vi "Bezier Spline.vi"(6 "positions":cluster{dbl[]}[](array[cluster]), 7 "Turn Rate":dbl=5.0 format="%#_13g", 8 "ending orientation (deg)":sgl=nan, 9 "starting orientation (deg)":sgl=nan, 10 "percision":sgl=0.01, 11 "waypts":cluster{"x":sgl, "y":sgl}[](array[cluster])) -> (0 "cubic spline ctrl pts":cluster{sgl, sgl}[][](array[cluster]), 1 "Tangents":cluster{sgl, sgl}[](array[cluster]), 2 "ctrl pts":cluster{sgl, sgl}[][](array[cluster]), 3 "bezier spline":cluster{"curve ":T1}[](array[cluster]), 4 "position out":sgl[][](array[numeric]))   [LabVIEW 2025]
uses:
  Types/Bezier Curve.ctl
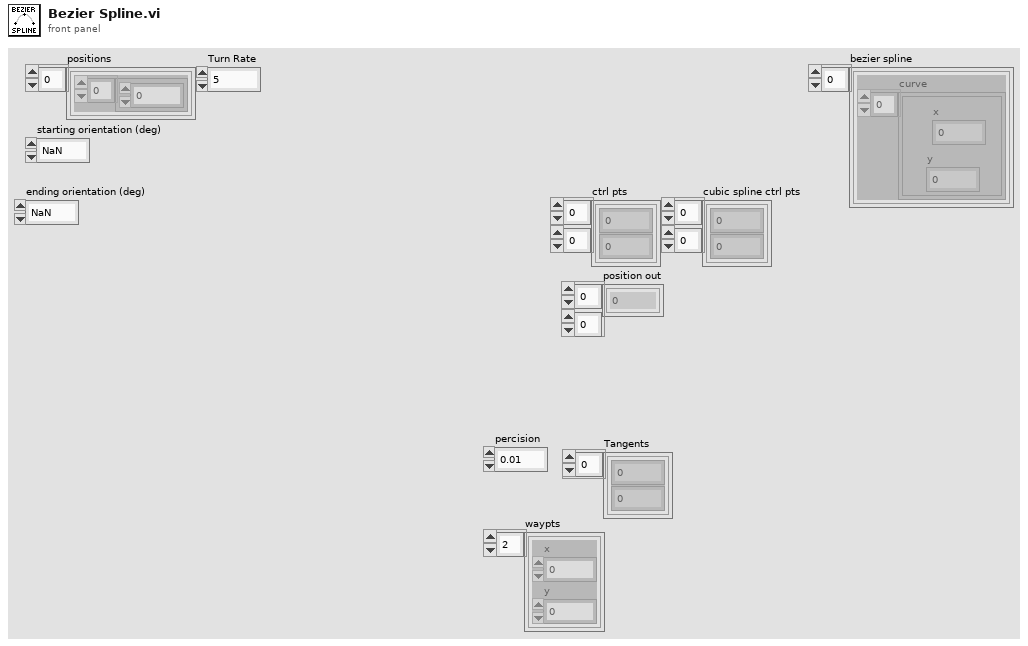
[diagram p1: front panel]
types:
  T1 = typedef "Bezier Curve.ctl" = cluster{"x":sgl, "y":sgl}[]
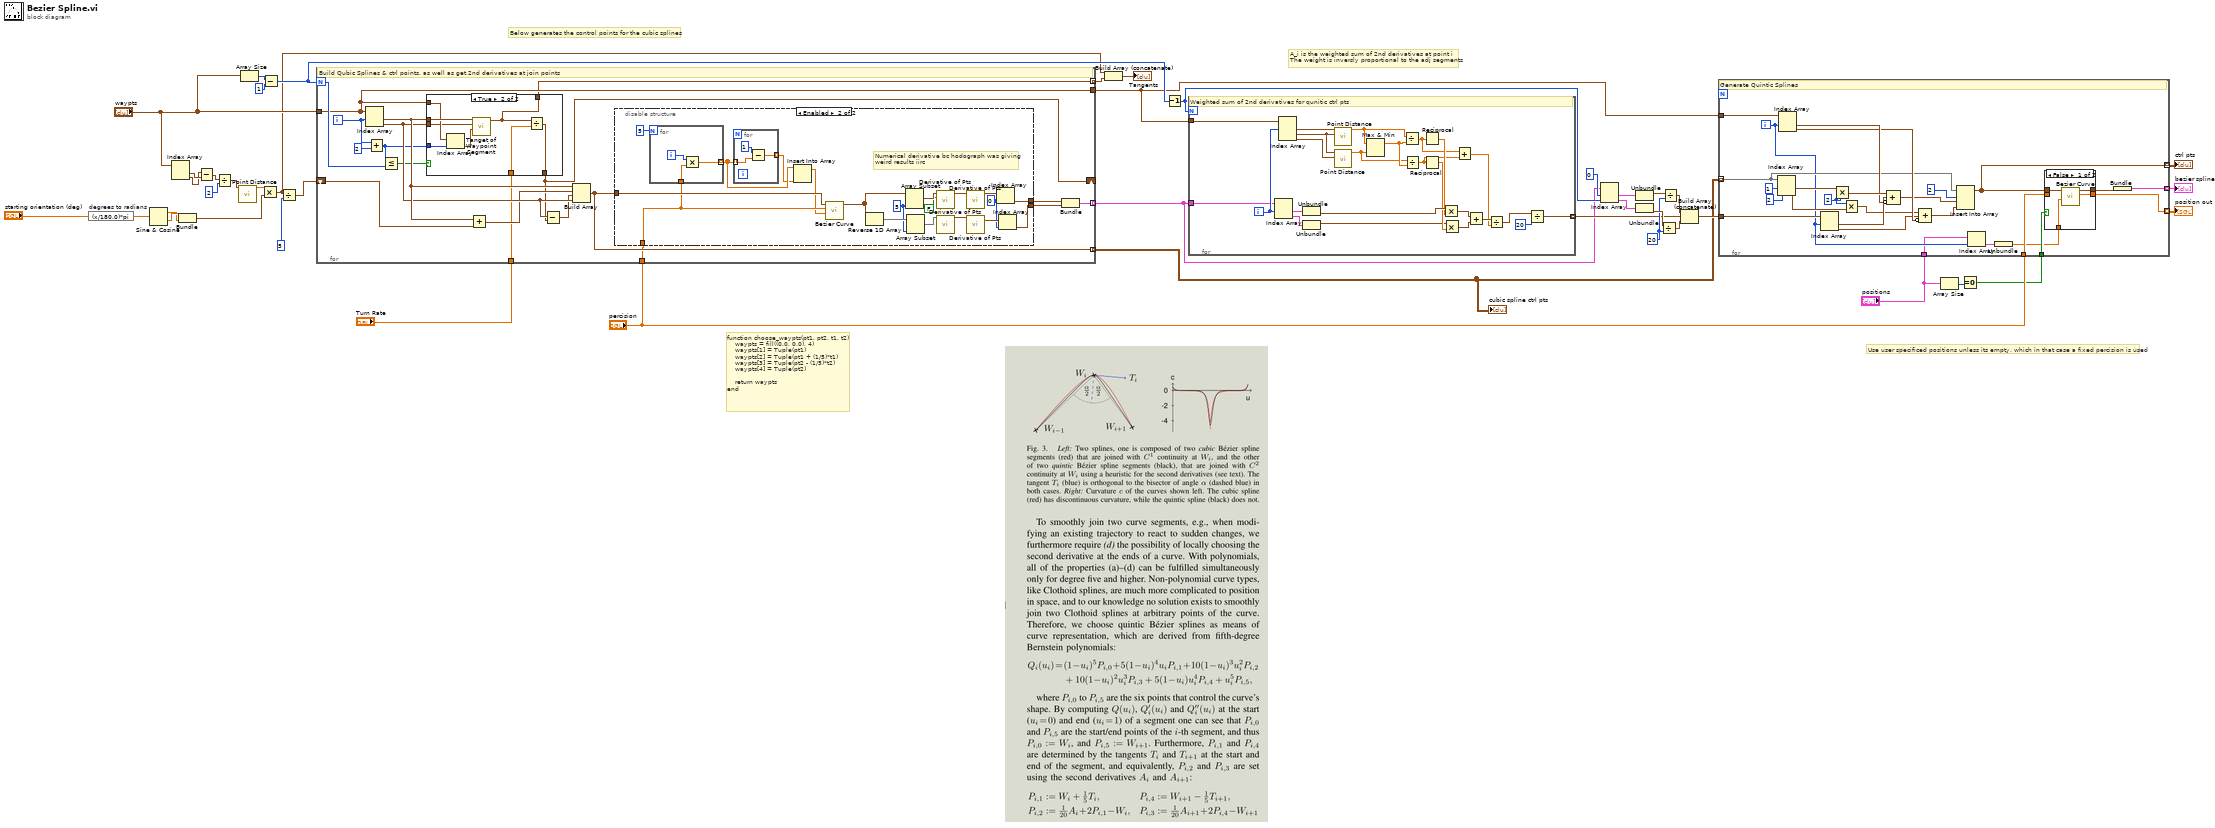
[diagram p0: block diagram]
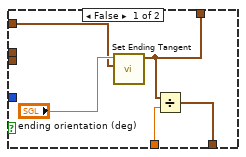
[diagram p2: hidden frame]
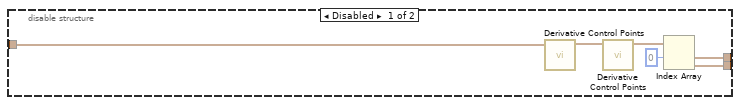
[diagram p3: hidden frame]
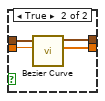
[diagram p4: hidden frame]
diagram:
  w26 = 20
  # "function choose_waypts(pt1, pt2, t1, t2)\n    waypts = fill((0.0, 0.0), 4)\n    waypts[1] = Tuple(pt1)\n    waypts[2] = Tuple(pt1 + (1/5)*t1)\n    waypts[3] = Tuple(pt2 - (1/5)*t2)\n    waypts[4] = Tuple(pt2)\n\n    return waypts\nend"
  # "Use user specificed positions unless its empty, which in that case a fixed percision is used"
  # "Below generates the control points for the cubic splines"
  # "A_i is the weighted sum of 2nd derivatives at point i\nThe weight is inversly proportional to the adj segments"
  n1 = expression code="(x/180.0)*pi" "degrees to radians"("starting orientation (deg)") -> (w16:sgl)
  n2 = Sine & Cosine(0:w16) -> (1:w14:sgl, 2:w15:sgl)
  n3 = Index Array(array="waypts") -> (element #1=w40:cluster{"x":sgl, "y":sgl}, element #2=w39:cluster{"x":sgl, "y":sgl})  [unwired: 2 in]
  n4 = Bundle(w15, w14) -> (w36:cluster{sgl, sgl})  [unwired: 1 in]
  n5 = Subtract(x=w39, y=w40) -> (x-y=w38:cluster{"x":sgl, "y":sgl})
  n6 = Divide(x=w38, y=u16 2) -> (x/y=w20:cluster{"x":sgl, "y":sgl})
  n7 = call "Point Distance.vi"("point a"=w20) -> ("dist"=w21:sgl)  [unwired: 10 in]
  n8 = Array Size(array="waypts") -> (size(s)=w42:i32)
  n9 = Multiply(x=w21, y=w36) -> (x*y=w10:cluster{sgl, sgl})
  n10 = Subtract(x=w42, y=1) -> (x-y=w35:i32)
  n11 = Divide(x=w10, y=5) -> (x/y=w18:cluster{sgl, sgl})
  n12 = for {
    N: w35 -> [w50]
    tunnel: "waypts" -> [w49]
    shift-right: [w48] -> _
    shift-left: w18 -> [w52]
    tunnel: [w47] -> w7 mode=indexing
    tunnel: [w55] -> w12 mode=indexing
    tunnel: [w49] -> w13
    tunnel: "percision" -> [w46]
    tunnel: [w45] -> w19 mode=indexing
    tunnel: "Turn Rate" -> [w43]
    i -> [w54]
    # "Build Qubic Splines & ctrl points, as well as get 2nd derivatives at join points"
    n13 = Index Array(array=w49, index #1=w54) -> (element #1=w61:cluster{"x":sgl, "y":sgl}, element #2=w60:cluster{"x":sgl, "y":sgl})  [unwired: 1 in]
    n14 = Add(x=w54, y=2) -> (x+y=w51:i32)
    n15 = Less Or Equal?(x=w51, y=w50) -> (x <= y?=w44:bool)
    n16 = case shown="True" w44 {
      tunnel: w61 -> [_ w74]
      tunnel: w60 -> [_ w69]
      tunnel: [w64 w73] -> w48
      tunnel: w51 -> [_ w72]
      tunnel: w49 -> [w65 w71]
      tunnel: [w63 w68] -> w45
      tunnel: w43 -> [w62 w67]
      frame False {
        n17 = call "Set Ending Tangent.vi"("waypts"=w65, "ending orientation"="ending orientation (deg)") -> ("ending tangent"=w63:cluster{sgl, sgl})  [unwired: 9 in]
        n18 = Divide(x=w63, y=w62) -> (x/y=w64:cluster{dbl, dbl})
      }
      frame True {
        n19 = Index Array(array=w71, index=w72) -> (element=w70:cluster{"x":sgl, "y":sgl})
        n20 = call "Tanget of Waypoint Segment.vi"("point c"=w70, "point b"=w69, "point a"=w74) -> ("T_i"=w68:cluster{sgl, sgl})  [unwired: 8 in]
        n21 = Divide(x=w68, y=w67) -> (x/y=w73:cluster{dbl, dbl})
      }
    }
    n22 = Add(x=w61, y=w52) -> (x+y=w59:cluster{dbl, dbl})
    n23 = Subtract(x=w60, y=w48) -> (x-y=w58:cluster{dbl, dbl})
    n24 = Build Array(w61, w59, w58, w60) -> (w47:cluster{"x":dbl, "y":dbl}[])
    n25 = disable-structure shown="Enabled" {
      disable-tunnel: w47 -> [w79 w87]
      disable-tunnel: [w76 w90] -> w57
      disable-tunnel: [w75 w89] -> w56
      disable-tunnel: w46 -> [_ w85]
      frame Disabled {
        n26 = call "Derivative Control Points.vi"("ctrl points"=w79) -> ("d ctrl pts"=w80:cluster{dbl, dbl}[])  [unwired: 10 in]
        n27 = call "Derivative Control Points.vi"("ctrl points"=w80) -> ("d ctrl pts"=w78:cluster{dbl, dbl}[])  [unwired: 10 in]
        n28 = Index Array(array=w78, index #1=0 ("index")) -> (element #1=w76:cluster{dbl, dbl}, element #2=w75:cluster{dbl, dbl})  [unwired: 1 in]
      }
      frame Enabled {
        w92 = 0 ("index")
        w91 = 5 ("length")
        # "Numerical derivative bc hodograph was giving\nweird results iirc"
        n29 = for {
          N: 5 -> [_]
          tunnel: w85 -> [w104]
          tunnel: [w103] -> w82 mode=indexing
          i -> [w105]
          n30 = Multiply(x=w105, y=w104) -> (x*y=w103:sgl)
        }
        n31 = for {
          tunnel: w82 -> [w102] mode=indexing
          tunnel: [w100] -> w81 mode=indexing
          n32 = Subtract(x=1 ("length"), y=w102) -> (x-y=w100:sgl)
        }
        n33 = Insert Into Array(array=w82, new element=w81) -> (w84:sgl[])  [unwired: 1 in]
        n34 = call "Bezier Curve.vi"("position"=w84, "percision"=w85, "ctrl points"=w87) -> ("curve"=w83:T1)  [unwired: 7 in, 1 out]
        n35 = Reverse 1D Array(array=w83) -> (reversed array=w99:T1)
        n36 = Array Subset(array=w83, length=w91) -> (w98:T1)  [unwired: 1 in]
        n37 = Array Subset(array=w99, length=w91) -> (w96:T1)  [unwired: 1 in]
        n38 = call "Derivative of Pts.vi"("pts"=w96) -> ("pts out"=w95:cluster{sgl, sgl}[])  [unwired: 10 in]
        n39 = call "Derivative of Pts.vi"("fix first pt?"=FALSE, "pts"=w98) -> ("pts out"=w97:cluster{sgl, sgl}[])  [unwired: 9 in]
        n40 = call "Derivative of Pts.vi"("pts"=w97) -> ("pts out"=w94:cluster{sgl, sgl}[])  [unwired: 10 in]
        n41 = call "Derivative of Pts.vi"("pts"=w95) -> ("pts out"=w93:cluster{sgl, sgl}[])  [unwired: 10 in]
        n42 = Index Array(array=w94, index=w92) -> (element=w90:cluster{sgl, sgl})
        n43 = Index Array(array=w93, index=w92) -> (element=w89:cluster{sgl, sgl})
      }
    }
    n44 = Bundle(w57, w56) -> (w55:cluster{cluster{sgl, sgl}, cluster{sgl, sgl}})  [unwired: 1 in]
  }
  "cubic spline ctrl pts" <- w7
  n45 = Build Array (concatenate)(w10, w19) -> (→"Tangents":cluster{sgl, sgl}[])
  n46 = Decrement(x=w35) -> (x-1=w30:i32)
  n47 = for {
    N: w30 -> [_]
    tunnel: w12 -> [w120]
    tunnel: w13 -> [w119]
    tunnel: [w109] -> w22 mode=indexing
    i -> [w129]
    # "Weighted sum of 2nd derivatives for qunitic ctrl pts"
    n48 = Index Array(array=w120, index #1=w129) -> (element #1=w128:cluster{cluster{sgl, sgl}, cluster{sgl, sgl}}, element #2=w127:cluster{cluster{sgl, sgl}, cluster{sgl, sgl}})  [unwired: 1 in]
    n49 = Index Array(array=w119, index #1=w129) -> (element #1=w126:cluster{"x":sgl, "y":sgl}, element #2=w125:cluster{"x":sgl, "y":sgl}, element #3=w124:cluster{"x":sgl, "y":sgl})  [unwired: 2 in]
    n50 = Unbundle(w128) -> (w117:cluster{sgl, sgl})  [unwired: 1 out]
    n51 = Unbundle(w127) -> (w114:cluster{sgl, sgl})  [unwired: 1 out]
    n52 = call "Point Distance.vi"("point b"=w125, "point a"=w126) -> ("dist"=w123:sgl)  [unwired: 9 in]
    n53 = call "Point Distance.vi"("point b"=w124, "point a"=w125) -> ("dist"=w121:sgl)  [unwired: 9 in]
    n54 = Max & Min(x=w123, y=w121) -> (max(x,y)=w122:sgl)  [unwired: 1 out]
    n55 = Divide(x=w123, y=w122) -> (x/y=w108:sgl)
    n56 = Divide(x=w121, y=w122) -> (x/y=w107:sgl)
    n57 = Reciprocal(x=w108) -> (1/x=w116:sgl)
    n58 = Reciprocal(x=w107) -> (1/x=w115:sgl)
    n59 = Multiply(x=w117, y=w116) -> (x*y=w113:cluster{sgl, sgl})
    n60 = Multiply(x=w114, y=w115) -> (x*y=w112:cluster{sgl, sgl})
    n61 = Add(x=w108, y=w107) -> (x+y=w106:sgl)
    n62 = Add(x=w113, y=w112) -> (x+y=w111:cluster{sgl, sgl})
    n63 = Divide(x=w111, y=w106) -> (x/y=w110:cluster{sgl, sgl})
    n64 = Divide(x=w110, y=20) -> (x/y=w109:cluster{sgl, sgl})
  }
  n65 = Index Array(array=w12, index #1=0 ("index"), index #2=w30) -> (element #1=w34:cluster{cluster{sgl, sgl}, cluster{sgl, sgl}}, element #2=w32:cluster{cluster{sgl, sgl}, cluster{sgl, sgl}})
  n66 = Unbundle(w34) -> (w27:cluster{sgl, sgl})  [unwired: 1 out]
  n67 = Unbundle(w32) -> (w29:cluster{sgl, sgl})  [unwired: 1 out]
  n68 = Divide(x=w29, y=w26) -> (x/y=w28:cluster{sgl, sgl})
  n69 = Divide(x=w27, y=w26) -> (x/y=w25:cluster{sgl, sgl})
  n70 = Build Array (concatenate)(w25, w22, w28) -> (w33:cluster{sgl, sgl}[])
  n71 = Array Size(array="positions") -> (size(s)=w8:i32)
  n72 = Equal To 0?(x=w8) -> (x = 0?=w5:bool)
  n73 = for {
    tunnel: w33 -> [w153]
    tunnel: w7 -> [w136] mode=indexing
    tunnel: w13 -> [w154]
    tunnel: "percision" -> [w140]
    tunnel: [w139] -> w24 mode=indexing
    tunnel: [w138] -> w9 mode=indexing
    tunnel: w5 -> [w137]
    tunnel: "positions" -> [w134]
    tunnel: [w130] -> w4 mode=indexing
    i -> [w135]
    w150 = u16 2
    # "Generate Quintic Splines"
    n74 = Index Array(array=w136, index #1=1 ("index"), index #2=2 ("index")) -> (element #1=w152:cluster{"x":dbl, "y":dbl}, element #2=w151:cluster{"x":dbl, "y":dbl})
    n75 = Index Array(array=w154, index #1=w135) -> (element #1=w147:cluster{"x":sgl, "y":sgl}, element #2=w146:cluster{"x":sgl, "y":sgl})  [unwired: 1 in]
    n76 = Index Array(array=w153, index #1=w135) -> (element #1=w148:cluster{sgl, sgl}, element #2=w144:cluster{sgl, sgl})  [unwired: 1 in]
    n77 = Multiply(x=w152, y=w150) -> (x*y=w149:cluster{"x":dbl, "y":dbl})
    n78 = Multiply(x=w150, y=w151) -> (x*y=w145:cluster{"x":dbl, "y":dbl})
    n79 = Compound Arithmetic op=ADD(w149, w148, invert w147) -> (w143:cluster{dbl, dbl})
    n80 = Compound Arithmetic op=ADD(w145, w144, invert w146) -> (w142:cluster{dbl, dbl})
    n81 = Insert Into Array(array=w136, index=2, new element #1=w143, new element #2=w142) -> (w139:cluster{"x":dbl, "y":dbl}[])
    n82 = Index Array(array=w134, index=w135) -> (element=w133:cluster{dbl[]})
    n83 = Unbundle(w133) -> (w132:dbl[])
    n84 = case shown="False" w137 {
      tunnel: w140 -> [_ w164]
      tunnel: [w159 w163] -> w131
      tunnel: w139 -> [w160 w162]
      tunnel: [w158 w161] -> w138
      tunnel: w132 -> [w157 _]
      frame False {
        n85 = call "Bezier Curve.vi"("position"=w157, "ctrl points"=w160) -> ("position out"=w158:sgl[], "curve"=w159:T1)  [unwired: 8 in]
      }
      frame True {
        n86 = call "Bezier Curve.vi"("percision"=w164, "ctrl points"=w162) -> ("position out"=w161:sgl[], "curve"=w163:T1)  [unwired: 8 in]
      }
    }
    n87 = Bundle("curve"=w131) -> (w130:cluster{"curve ":T1})  [unwired: 1 in]
  }
  "ctrl pts" <- w24
  "position out" <- w9
  "bezier spline" <- w4
